vi "while_v0_v10.vi"() -> ()   [LabVIEW 2009]
panel:
  in  "stop":bool
  out "Waveform Chart":dbl(graph)=0.6409697683959468
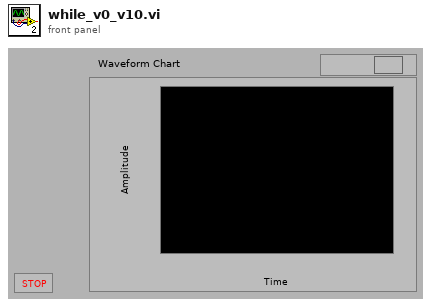
[diagram p1: front panel]
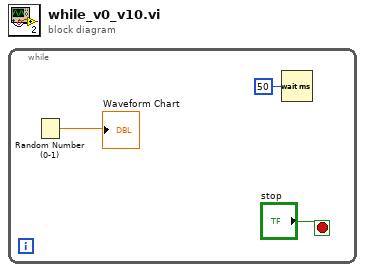
[diagram p0: block diagram]
diagram:
  n1 = while {
    stop <- "stop" stop-if-true
    n2 = Random Number (0-1)() -> (number: 0 to 1=→"Waveform Chart":dbl)
    n3 = Wait (ms)(milliseconds to wait=u32 50) -> ()  [unwired: 1 out]
  }
